vi "ReplaceMe.vi"(11 "In":variant) -> (3 "Out":variant)   [LabVIEW 2018]
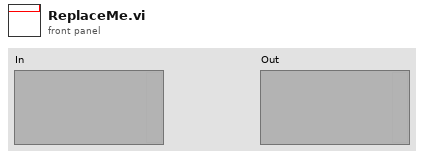
[diagram p1: front panel]
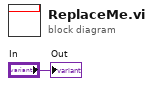
[diagram p0: block diagram]
diagram:
  "Out" <- "In"
